vi "AO Python Write Read TCP Data.vi"(0 "Connection ID":refnum<k5>, 7 "Write String":string, 11 "Error":errorcluster, 13 "Timeout (ms)":i32=5000) -> (4 "Connection ID (Dup)":refnum<k5>, 8 "Read String":string, 15 "Error Out":errorcluster)   [LabVIEW 2016]
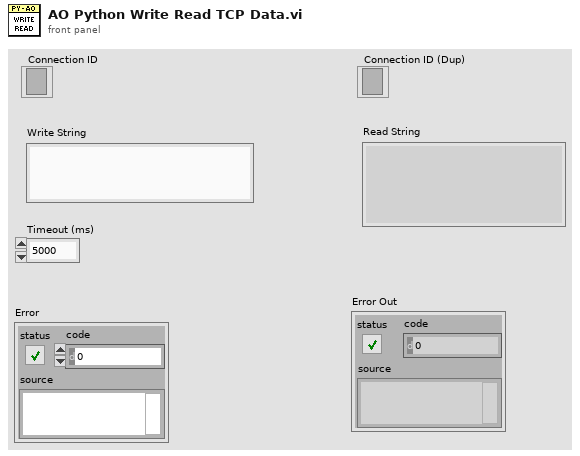
[diagram p1: front panel]
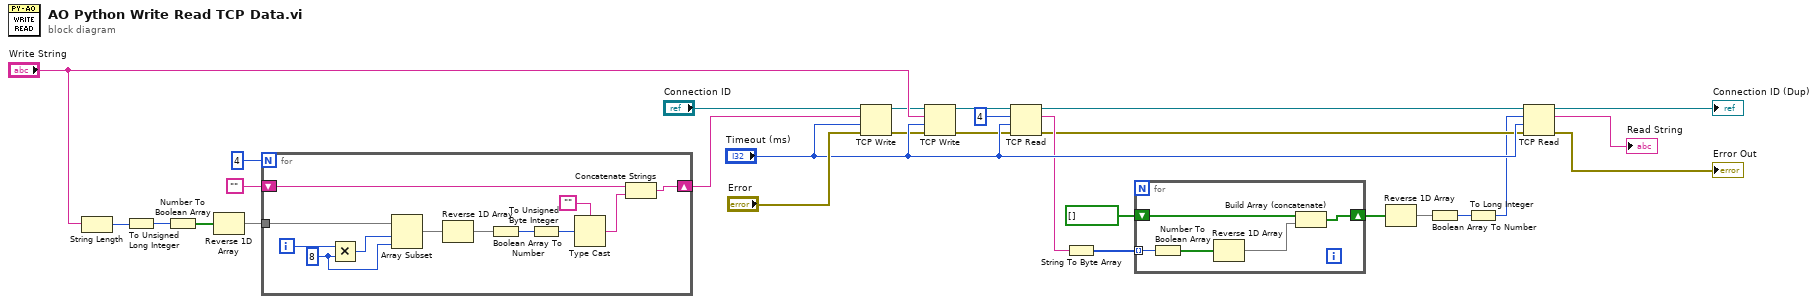
[diagram p0: block diagram]
diagram:
  n1 = String Length(string="Write String") -> (length=w28:i32)
  n2 = To Unsigned Long Integer(number=w28) -> (unsigned 32bit integer=w27:u32)
  n3 = Number To Boolean Array(number=w27) -> (Boolean array=w20:bool[])
  n4 = Reverse 1D Array(array=w20) -> (reversed array=w19:bool[])
  n5 = for {
    N: 4 -> [_]
    tunnel: w19 -> [w40]
    shift-right: [w33] -> w24
    shift-left: "" -> [w34]
    i -> [w39]
    w37 = 8 ("y")
    n6 = Multiply(x=w39, y=w37) -> (x*y=w38:i32)
    n7 = Array Subset(array=w40, index=w38, length=w37) -> (w36:bool[])
    n8 = Reverse 1D Array(array=w36) -> (reversed array=w29:bool[])
    n9 = Boolean Array To Number(Boolean array=w29) -> (number=w32:u32)
    n10 = To Unsigned Byte Integer(number=w32) -> (unsigned 8bit integer=w30:u8)
    n11 = Type Cast(type="", x=w30) -> (*(type *) &x=w31:string)
    n12 = Concatenate Strings(w34, w31) -> (w33:string)
  }
  n13 = TCP Write(connection ID="Connection ID", data in=w24, error in (no error)="Error", 9:"Timeout (ms)") -> (connection ID out=w17:refnum<k5>, error out=w16:errorcluster)  [unwired: 1 out]
  n14 = TCP Write(connection ID=w17, data in="Write String", error in (no error)=w16, 9:"Timeout (ms)") -> (connection ID out=w15:refnum<k5>, error out=w14:errorcluster)  [unwired: 1 out]
  n15 = TCP Read(connection ID=w15, bytes to read=4, error in (no error)=w14, 9:"Timeout (ms)") -> (connection ID out=w4:refnum<k5>, data out=w9:string, error out=w3:errorcluster)  [unwired: 1 in]
  n16 = String To Byte Array(string=w9) -> (unsigned byte array=w8:u8[])
  n17 = for {
    tunnel: w8 -> [w45] mode=indexing
    shift-right: [w42] -> w6
    shift-left: bool[] [] -> [w44]
    n18 = Number To Boolean Array(number=w45) -> (Boolean array=w43:bool[])
    n19 = Reverse 1D Array(array=w43) -> (reversed array=w41:bool[])
    n20 = Build Array (concatenate)(w44, w41) -> (w42:bool[])
  }
  n21 = Reverse 1D Array(array=w6) -> (reversed array=w1:bool[])
  n22 = Boolean Array To Number(Boolean array=w1) -> (number=w5:u32)
  n23 = To Long Integer(number=w5) -> (32bit integer=w2:i32)
  n24 = TCP Read(connection ID=w4, bytes to read=w2, error in (no error)=w3, 9:"Timeout (ms)") -> (connection ID out=→"Connection ID (Dup)":refnum<k5>, data out=→"Read String":string, error out=→"Error Out":errorcluster)  [unwired: 1 in]
